vi "Cleanup.vi"(7 "Close Engine? (T)":bool=TRUE, 8 "error in (no error)":errorcluster, 11 "TSnax UI Manager in":refnum<class "TSnax UI Manager.lvclass">) -> (0 "error out":errorcluster)   [LabVIEW 2020, in "TSnax UI.lvlib" / "TSnax UI Manager.lvclass"]
uses:
  TSnax UI Manager.lvclass
  TSnax UI Manager.lvclass/TSnax UI Manager.ctl
  <vilib>/IlluminatedG/IG OOPanel/OOPanel/Manager/Manager.lvclass
  TSnax/Engine/Engine.lvclass
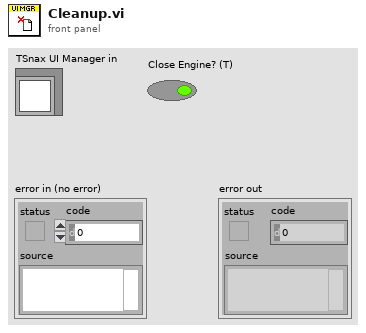
[diagram p1: front panel]
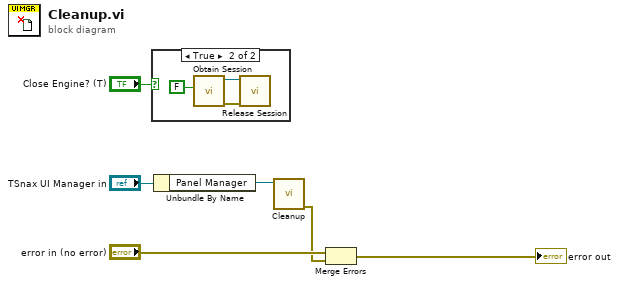
[diagram p0: block diagram]
diagram:
  n1 = case shown="True" "Close Engine? (T)" {
    frame False {
    }
    frame True {
      n2 = call "Obtain Session.vi"("Create if needed? (T)"=FALSE) -> ("error out"=w8:errorcluster, "Engine out"=w7:refnum<class "Engine.lvclass">)  [unwired: 9 in]
      n3 = call "Release Session.vi"("error in (no error)"=w8, "Engine in"=w7) -> ()  [unwired: 9 in, 1 out]
    }
  }
  n4 = Unbundle By Name("TSnax UI Manager in") -> ("Panel Manager"=w4:refnum<class "Manager.lvclass">)
  n5 = call <vilib>:"Cleanup.vi"("Manager in"=w4) -> ("error out"=w2:errorcluster)  [unwired: 8 in, 2 out]
  n6 = Merge Errors("error in (no error)", w2) -> (→"error out":errorcluster)
